vi "Kicker.vi"(7 "Mode":T4, 8 "error in (no error)":errorcluster, 9 "Default Position":bool, 10 "State":bool, 11 "SolenoidDevRef":T1={"DevStatus"={"status"=FALSE, "code"=0, "source"=""}, "Solenoid Module"=enum."Solenoid Module 1", "Forward Solenoid Channel"=enum."Invalid", "Reverse Solenoid Channel"=enum."Invalid"}) -> (0 "error out":errorcluster)   [LabVIEW 2013]
doc: "Takes in button value from toggle indicator. If toggle indicator is T, it takes the opposite value of DefaultPosition."
uses:
  PnuematicMode.ctl
  <vilib>/Rock Robotics/WPI/Solenoid/WPI_SolenoidDevRef.ctl
  <vilib>/Rock Robotics/SystemInterfaces/Typedef/FPGA_TypedefSolenoidModule.ctl
  <vilib>/Rock Robotics/WPI/Solenoid/WPI_SolenoidChannel.ctl
  <vilib>/Rock Robotics/WPI/Solenoid/WPI_SolenoidValue.ctl
  <vilib>/Rock Robotics/WPI/Solenoid/WPI_SolenoidSetEnum.vi
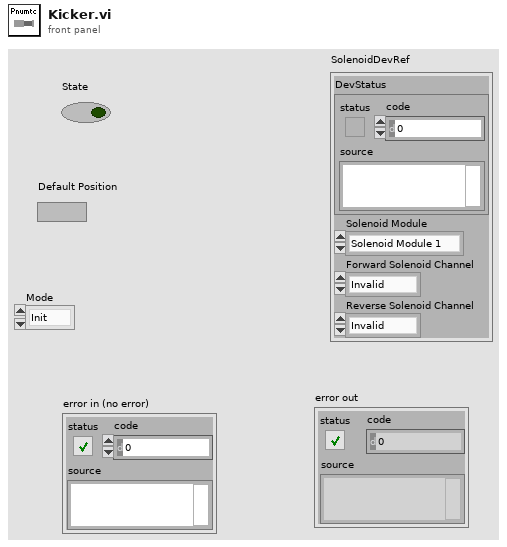
[diagram p1: front panel]
types:
  T1 = typedef "WPI_SolenoidDevRef.ctl" = cluster{"DevStatus":errorcluster, "Solenoid Module":T2, "Forward Solenoid Channel":T3, "Reverse Solenoid Channel":T3}
  T2 = typedef "FPGA_TypedefSolenoidModule.ctl" = enum16{"Solenoid Module 1", "Solenoid Module 2"}
  T3 = typedef "WPI_SolenoidChannel.ctl" = enum8{"Solenoid 1", "Solenoid 2", "Solenoid 3", "Solenoid 4", "Solenoid 5", "Solenoid 6", "Solenoid 7", "Solenoid 8", "Invalid"}
  T4 = typedef "PnuematicMode.ctl" = enum16{"Init", "SetState", "Disable"}
  T5 = typedef "WPI_SolenoidValue.ctl" = enum16{"Off", "On", "Forward", "Reverse"}
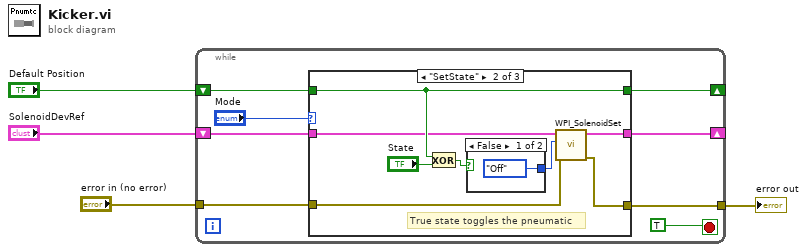
[diagram p0: block diagram]
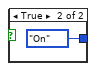
[diagram p3: hidden frame]
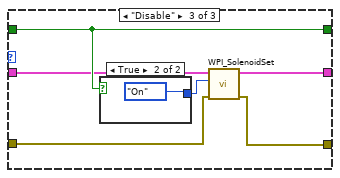
[diagram p4: hidden frame]
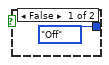
[diagram p5: hidden frame]
diagram:
  n1 = while {
    shift-right: [w10] -> _
    shift-left: "Default Position" -> [w12]
    shift-right: [w8] -> _
    shift-left: "SolenoidDevRef" -> [w7]
    tunnel: "error in (no error)" -> [w6]
    tunnel: [w5] -> w1
    stop <- TRUE stop-if-true
    n2 = case shown="\"SetState\"" "Mode" {
      tunnel: w12 -> [w15 w22 w30]
      tunnel: [w15 w22 w30] -> w10
      tunnel: [w14 w18 w28] -> w8
      tunnel: w7 -> [w14 w19 w29]
      tunnel: w6 -> [w13 w17 w27]
      tunnel: [w13 w16 w26] -> w5
      frame "Init", Default {
      }
      frame "SetState" {
        # "True state toggles the pneumatic"
        n3 = Exclusive Or(1:"State", 2:w22) -> (0:w21:bool)
        n4 = case shown="False" w21 {
          tunnel: [WPI_SolenoidValue."Off" ("Value") WPI_SolenoidValue."On" ("Value")] -> w20
          frame False {
          }
          frame True {
          }
        }
        n5 = call-poly <vilib>:"WPI_SolenoidSet.vi"("error in (no error)"=w17, "Value"=w20, "SolenoidDevRef"=w19) -> ("error out"=w16:errorcluster, "SolenoidDevRef"=w18:T1)  [unwired: 7 in]
      }
      frame "Disable" {
        n6 = case shown="True" w30 {
          tunnel: [WPI_SolenoidValue."Off" ("Value") WPI_SolenoidValue."On" ("Value")] -> w31
          frame False {
          }
          frame True {
          }
        }
        n7 = call-poly <vilib>:"WPI_SolenoidSet.vi"("error in (no error)"=w27, "Value"=w31, "SolenoidDevRef"=w29) -> ("error out"=w26:errorcluster, "SolenoidDevRef"=w28:T1)  [unwired: 7 in]
      }
    }
  }
  "error out" <- w1
